vi "getCCT.vi"(4 "Fiber Num":i32, 6 "Error":bool, 7 "VISA resource name":refnum<visa-resource-name>="ASRL13::INSTR") -> (0 "DELTA-UV":dbl, 1 "CCT":u32, 2 "Error":bool, 3 "dup VISA resource name":refnum<visa-resource-name>="ASRL13::INSTR")   [LabVIEW 2018]
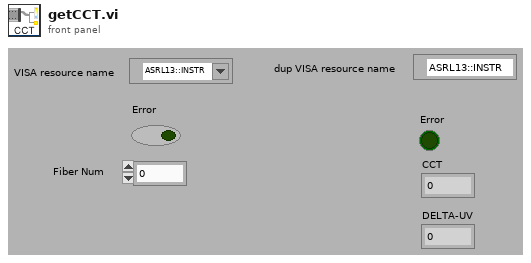
[diagram p1: front panel]
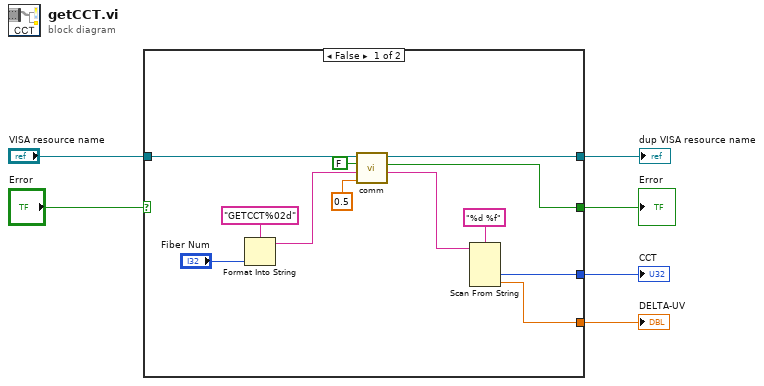
[diagram p0: block diagram]
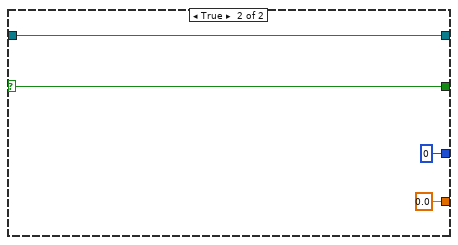
[diagram p2: hidden frame]
diagram:
  n1 = case shown="False" "Error" {
    selector: "Error" -> [_ w21]
    tunnel: "VISA resource name" -> [w18 w22]
    tunnel: [w10 u32 0] -> w5
    tunnel: [w9 0.0] -> w4
    tunnel: [w8 w22] -> w2
    tunnel: [w7 w21] -> w1
    frame False {
      n2 = Format Into String(format string="GETCCT%02d" ("Substring"), "Fiber Num") -> (resulting string=w15:string)  [unwired: 2 in, 1 out]
      n3 = call "comm.vi"("Timeout (s)"=0.5, "Command"=w15, "Error"=FALSE, "VISA resource name"=w18) -> ("Response"=w12:string, "Error"=w7:bool, "dup VISA resource name"=w8:refnum<visa-resource-name>)  [unwired: 2 in, 1 out]
      n4 = Scan From String(format string="%d %f", input string=w12) -> (output 1=w10:i32, output 2=w9:dbl)  [unwired: 4 in, 3 out]
    }
    frame True {
    }
  }
  "CCT" <- w5
  "DELTA-UV" <- w4
  "Error" <- w1
  "dup VISA resource name" <- w2
